vi "Enter.vi"(8 "error in (no error)":errorcluster, 11 "Wall in":refnum<class "Wall.lvclass">) -> (0 "error out":errorcluster, 3 "Wall out":refnum<class "Wall.lvclass">)   [LabVIEW 2016, in "Wall.lvclass"]
uses:
  Wall.lvclass
  MapSite/MapSite.lvclass
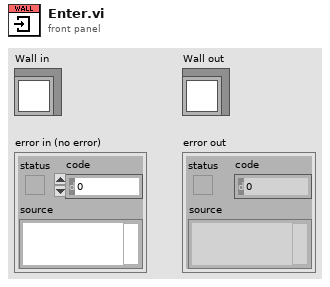
[diagram p1: front panel]
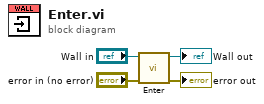
[diagram p0: block diagram]
diagram:
  n1 = call-parent "Enter.vi"("error in (no error)"="error in (no error)", "MapSite in"="Wall in") -> ("error out"=→"error out":errorcluster, "MapSite out"=→"Wall out":refnum<class "Wall.lvclass">)  [unwired: 8 in]
